vi "List All Nodes MAC.vi"() -> (2 "Nodes Short ID":string[](array[string]), 3 "Nodes MAC List":string[](array[string]))   [LabVIEW 2013, in "ZDAQ.lvlib"]
uses:
  ZDAQ.lvlib
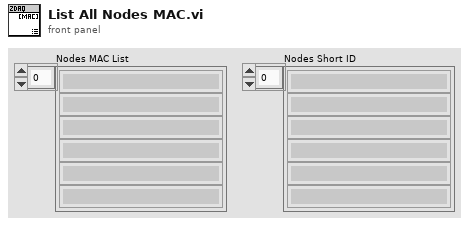
[diagram p1: front panel]
types:
  T1 = cluster{"Device Type":enum16{"Coordinator", "Router", "Device"}, "ID":string, "DeviceName":string, "Short NodeID":string, "Long NodeID":string}
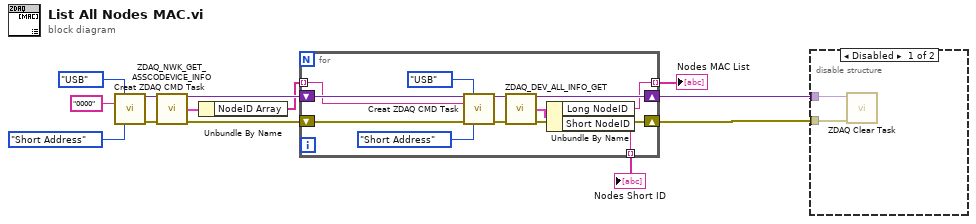
[diagram p0: block diagram]
diagram:
  n1 = call <userlib>:"Creat ZDAQ CMD Task.vi"("GatewayType"=enum16{"USB", "Ethernet"}."USB", "NodeID"="0000" ("EthernetIP"), "NodeID Type"=enum16{"Long Address", "Short Address"}."Short Address") -> ("Task Out"=w11:variant, "error out"=w10:errorcluster)  [unwired: 11 in]
  n2 = call <userlib>:"ZDAQ_NWK_GET_ASSCODEVICE_INFO.vi"("Task In"=w11, "error in (no error)"=w10) -> ("Task Out"=w8:variant, "Nwk Nodes Info"=w6:cluster{"Numbers":u32, "NodeID Array":string[]}, "error out"=w9:errorcluster)  [unwired: 10 in, 1 out]
  n3 = Unbundle By Name(w6) -> ("NodeID Array"=w2:string[])
  n4 = for {
    shift-right: [w18] -> w4
    shift-left: w9 -> [w25]
    shift-right: [w19] -> w5
    shift-left: w8 -> [w24]
    tunnel: [w16] -> w3 mode=indexing
    tunnel: w2 -> [w15] mode=indexing
    tunnel: [w14] -> w1 mode=indexing
    n5 = call <userlib>:"Creat ZDAQ CMD Task.vi"("Task In"=w24, "GatewayType"=enum16{"USB", "Ethernet"}."USB", "NodeID"=w15, "error in (no error)"=w25, "NodeID Type"=enum16{"Long Address", "Short Address"}."Short Address") -> ("Task Out"=w21:variant, "error out"=w20:errorcluster)  [unwired: 9 in]
    n6 = call <userlib>:"ZDAQ_DEV_ALL_INFO_GET.vi"("Task In"=w21, "error in (no error)"=w20) -> ("Task Out"=w19:variant, "Device Info"=w17:T1, "error out"=w18:errorcluster)  [unwired: 10 in, 1 out]
    n7 = Unbundle By Name(w17) -> ("Long NodeID"=w16:string, "Short NodeID"=w14:string)
  }
  "Nodes MAC List" <- w3
  "Nodes Short ID" <- w1
  n8 = disable-structure shown="Disabled" {
    disable-tunnel: w5 -> [w27 _]
    disable-tunnel: w4 -> [w26 _]
    frame Disabled {
      n9 = call <userlib>:"ZDAQ Clear Task.vi"("error in (no error)"=w26, "Task In"=w27) -> ()  [unwired: 8 in, 2 out]
    }
    frame Enabled {
    }
  }
